vi "LabVIEW Dependencies Path.vi"(11 "error in (no error)":errorcluster) -> (4 "MeasLink Path":path, 6 "Arrange BD Path":path, 8 "Arrange FP Path":path, 15 "error out":errorcluster)   [LabVIEW 2021, in "Path Functions.lvlib"]
uses:
  Path Functions.lvlib
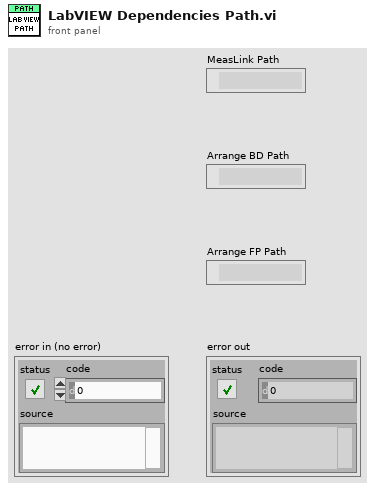
[diagram p1: front panel]
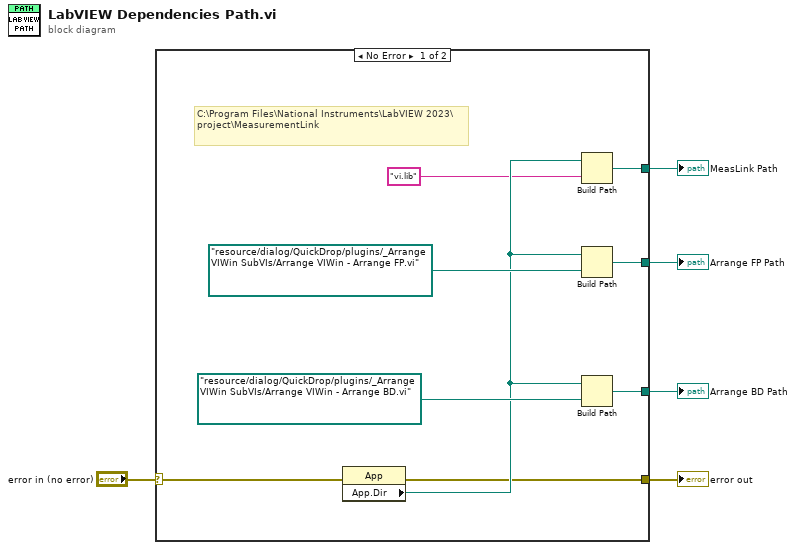
[diagram p0: block diagram]
diagram:
  n1 = case shown="No Error" "error in (no error)" {
    selector: "error in (no error)" -> [w7 w15]
    tunnel: [w10 _] -> w5
    tunnel: [w9 _] -> w4
    tunnel: [w8 _] -> w3
    tunnel: [w6 w15] -> w1
    frame No Error {
      # "C:\\Program Files\\National Instruments\\LabVIEW 2023\\project\\MeasurementLink"
      n2 = property class="App"(error in=w7) -> (error out=w6:errorcluster, "App.Dir"=w12:path)  [unwired: 1 in, 1 out]
      n3 = Build Path(base path=w12, name or relative path="vi.lib" ("string")) -> (appended path=w10:path)
      n4 = Build Path(base path=w12, name or relative path=path "resource/dialog/QuickDrop/plugins/_Arrange VIWin SubVIs/Arrange VIWin - Arrange FP.vi") -> (appended path=w9:path)
      n5 = Build Path(base path=w12, name or relative path=path "resource/dialog/QuickDrop/plugins/_Arrange VIWin SubVIs/Arrange VIWin - Arrange BD.vi") -> (appended path=w8:path)
    }
    frame Error {
    }
  }
  "MeasLink Path" <- w5
  "Arrange FP Path" <- w4
  "Arrange BD Path" <- w3
  "error out" <- w1
